vi "Write Categories.vi"(8 "error in (no error)":errorcluster, 10 "Categories":refnum<data-value>, 11 "VIStore in":refnum<class "VIStore.lvclass">) -> (0 "error out":errorcluster, 3 "VIStore out":refnum<class "VIStore.lvclass">)   [LabVIEW 2015, in "VI App Store.lvlib" / "VIStore.lvclass"]
uses:
  VIStore.lvclass
  Classes/Category/Category.lvclass
  VIStore.lvclass/VIStore.ctl
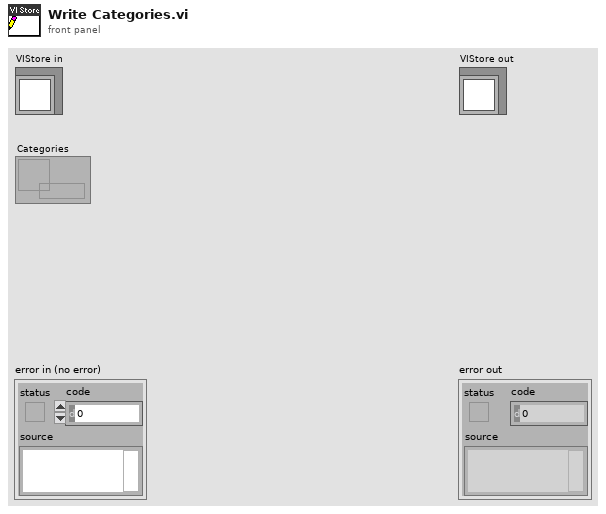
[diagram p1: front panel]
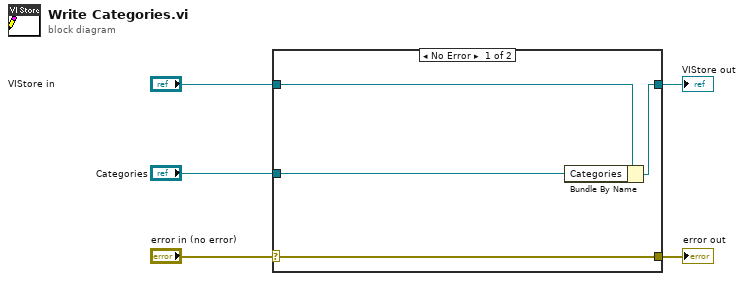
[diagram p0: block diagram]
diagram:
  n1 = case shown="No Error" "error in (no error)" {
    selector: "error in (no error)" -> [w9 w10]
    tunnel: [w9 w10] -> w4
    tunnel: [w7 w11] -> w2
    tunnel: "VIStore in" -> [w8 w11]
    tunnel: "Categories" -> [w6 _]
    frame No Error {
      n2 = Bundle By Name(cluster=w8, "Categories"=w6) -> (w7:refnum<class "VIStore.lvclass">)
    }
    frame Error {
    }
  }
  "error out" <- w4
  "VIStore out" <- w2
